vi "Read Address.vi"(8 "error in":errorcluster, 11 "Alicat in":refnum<class "Alicat.lvclass">) -> (0 "error out":errorcluster, 2 "Address":string, 3 "Alicat out":refnum<class "Alicat.lvclass">)   [LabVIEW 2015, in "Alicat.lvlib" / "Alicat.lvclass"]
doc: "Read the address of the device (should be a single characterr A...Z)."
uses:
  Alicat.lvclass
  Alicat.lvclass/Alicat.ctl
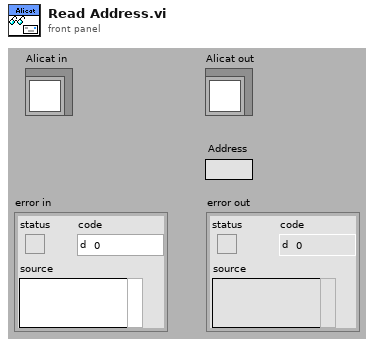
[diagram p1: front panel]
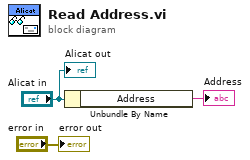
[diagram p0: block diagram]
diagram:
  n1 = Unbundle By Name("Alicat in") -> ("Address"=→"Address":string)
  "error out" <- "error in"
  "Alicat out" <- "Alicat in"
